vi "CCD Exposure Indicator V0.80.vi"(0 "ExpTime":dbl=4.0 format="%.2f") -> ()   [LabVIEW 2025]
doc: "Author: Scott Hannahs <sth@magnet.fsu.edu>\n\nThis software is licensed for use under the “MIT License\"\nCopyright (c) 2025 Scott Hannahs, sth@sth@magnet.sthnet.net\n\nPermission is hereby granted, free of charge, to any person obtaining a copy of this software and associated documentation files (the \"Software\"), to deal in the Software without restriction, including without limitation the rights to use, copy, modify, merge, publish, distribute, sublicense, and/or sell copies of the Software, and to permit persons to whom the Software is furnished to do so, subject to the following conditions: The above copyright notice and this permission notice shall be included in all copies or substantial portions of the Software.\n\nTHE SOFTWARE IS PROVIDED \"AS IS\", WITHOUT WARRANTY OF ANY KIND, EXPRESS OR IMPLIED, INCLUDING BUT NOT LIMITED TO THE WARRANTIES OF MERCHANTABILITY, FITNESS FOR A PARTICULAR PURPOSE AND NONINFRINGEMENT. IN NO EVENT SHALL THE AUTHORS OR COPYRIGHT HOLDERS BE LIABLE FOR ANY CLAIM, DAMAGES OR OTHER LIABILITY, WHETHER IN AN ACTION OF CONTRACT, TORT OR OTHERWISE, ARISING FROM, OUT OF OR IN CONNECTION WITH THE SOFTWARE OR THE USE OR OTHER DEALINGS IN THE SOFTWARE."
uses:
  Globals and TypeDefs/Global Varibal Control.vi
panel:
  out "x-y":u32
  out "Exp flash":string caption="Exposure"
  out "Exposure":dbl(slide)=0.133 scale=0.0..3.0 scale format="%.1f"
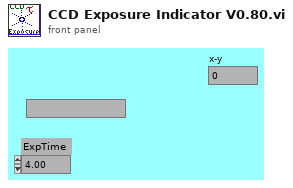
[diagram p1: front panel]
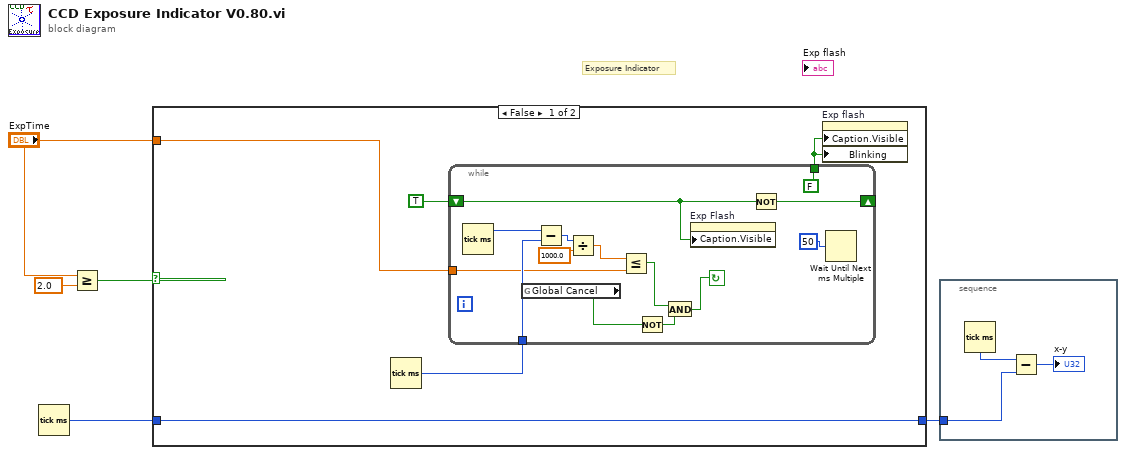
[diagram p0: block diagram]
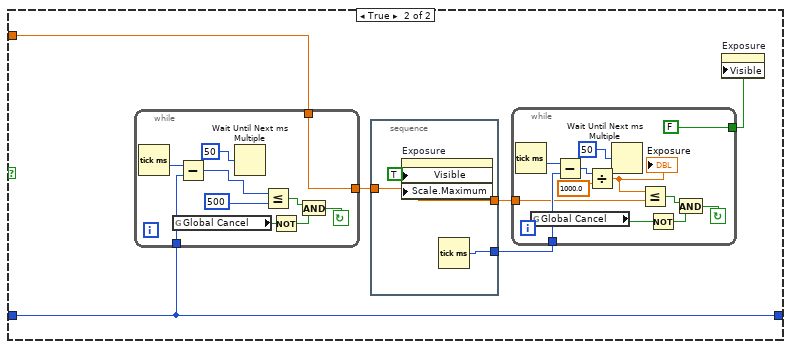
[diagram p2: hidden frame]
diagram:
  # "Exposure Indicator"
  n1 = Tick Count (ms)() -> (millisecond timer value=w2:u32)
  n2 = Greater Or Equal?(x="ExpTime", y=2.0) -> (x >= y?=w5:bool)
  n3 = case shown="False" w5 {
    tunnel: "ExpTime" -> [w7 w26]
    tunnel: [w6 w27] -> w1
    tunnel: w2 -> [w6 w27]
    frame False {
      n4 = Tick Count (ms)() -> (millisecond timer value=w10:u32)
      n5 = while {
        shift-left: TRUE ("Visible") -> [w15]
        shift-right: [w16] -> _
        tunnel: [FALSE ("Visible")] -> w9
        tunnel: w7 -> [w17]
        tunnel: w10 -> [w21]
        stop <- w12 continue-if-true
        n6 = Tick Count (ms)() -> (millisecond timer value=w23:u32)
        n7 = global read "Global Varibal Control.vi" "Global Cancel"() -> (w11:bool)
        n8 = Subtract(x=w23, y=w21) -> (x-y=w22:u32)
        n9 = Divide(x=w22, y=1000.0) -> (x/y=w18:dbl)
        n10 = Less Or Equal?(x=w18, y=w17) -> (x <= y?=w13:bool)
        n11 = Not(x=w11) -> (.not. x?=w14:bool)
        n12 = And(x=w13, y=w14) -> (x .and. y?=w12:bool)
        n13 = property on="Exp Flash" class="Str"("Caption.Visible"=w15) -> ()  [unwired: 2 in, 2 out]
        n14 = Not(x=w15) -> (.not. x?=w16:bool)
        n15 = Wait Until Next ms Multiple(millisecond multiple=u32 50) -> ()  [unwired: 1 out]
      }
      n16 = property on="Exp flash" class="Str"("Caption.Visible"=w9, "Blinking"=w9) -> ()  [unwired: 2 in, 2 out]
    }
    frame True {
      n17 = while {
        tunnel: [w45] -> w25
        tunnel: w26 -> [w45]
        tunnel: w27 -> [w44]
        stop <- w48 continue-if-true
        n18 = Tick Count (ms)() -> (millisecond timer value=w52:u32)
        n19 = global read "Global Varibal Control.vi" "Global Cancel"() -> (w43:bool)
        n20 = Subtract(x=w52, y=w44) -> (x-y=w47:u32)
        n21 = Wait Until Next ms Multiple(millisecond multiple=u32 50) -> ()  [unwired: 1 out]
        n22 = Less Or Equal?(x=w47, y=u32 500 ("millisecond multiple")) -> (x <= y?=w49:bool)
        n23 = Not(x=w43) -> (.not. x?=w50:bool)
        n24 = And(x=w49, y=w50) -> (x .and. y?=w48:bool)
      }
      n25 = stacked-sequence {
        tunnel: [w54] -> w30
        tunnel: w25 -> [w53]
        tunnel: [w53] -> w29
        frame #0 {
          n26 = property on="Exposure" class="Slide (strict)"("Visible"=TRUE, "Scale.Maximum"=w53) -> ()  [unwired: 2 in, 2 out]
          n27 = Tick Count (ms)() -> (millisecond timer value=w54:u32)
        }
      }
      n28 = while {
        tunnel: [FALSE ("Visible")] -> w28
        tunnel: w29 -> [w37]
        tunnel: w30 -> [w39]
        stop <- w32 continue-if-true
        n29 = Tick Count (ms)() -> (millisecond timer value=w41:u32)
        n30 = global read "Global Varibal Control.vi" "Global Cancel"() -> (w31:bool)
        n31 = Subtract(x=w41, y=w39) -> (x-y=w40:u32)
        n32 = Divide(x=w40, y=1000.0) -> (x/y=w36:dbl)
        "Exposure" <- w36
        n33 = Wait Until Next ms Multiple(millisecond multiple=u32 50) -> ()  [unwired: 1 out]
        n34 = Less Or Equal?(x=w36, y=w37) -> (x <= y?=w33:bool)
        n35 = Not(x=w31) -> (.not. x?=w34:bool)
        n36 = And(x=w33, y=w34) -> (x .and. y?=w32:bool)
      }
      n37 = property on="Exposure" class="Slide (strict)"("Visible"=w28) -> ()  [unwired: 2 in, 2 out]
    }
  }
  n38 = stacked-sequence {
    tunnel: w1 -> [w58]
    frame #0 {
      n39 = Tick Count (ms)() -> (millisecond timer value=w57:u32)
      n40 = Subtract(x=w57, y=w58) -> (x-y=→"x-y":u32)
    }
  }
